vi "SCI_Rx_Pack.vi"(6 "确认":bool, 8 "SCI RX数据块":u16[](array[numeric]) format="%x") -> (3 "SciPckOut":T1={"包头"=170, "数据低8位"=0, "数据低高8位"=0, "数据类型"=0, "CRC余数"=0, "数据无效"=FALSE, "数据更新"=FALSE} {"包头" format="%02x"; "数据低8位" format="%02x"; "数据低高8位" format="%02x"; "数据类型" items=["VOID"]; "CRC余数" format="%02x"}, 5 "读数据块":u16[](array[numeric]) format="%x")   [LabVIEW 2015]
uses:
  SCI_DataPck.ctl
  SCI_DataType.ctl
  SCI_FrameIndex.ctl
  SCI_FrameNumber.ctl
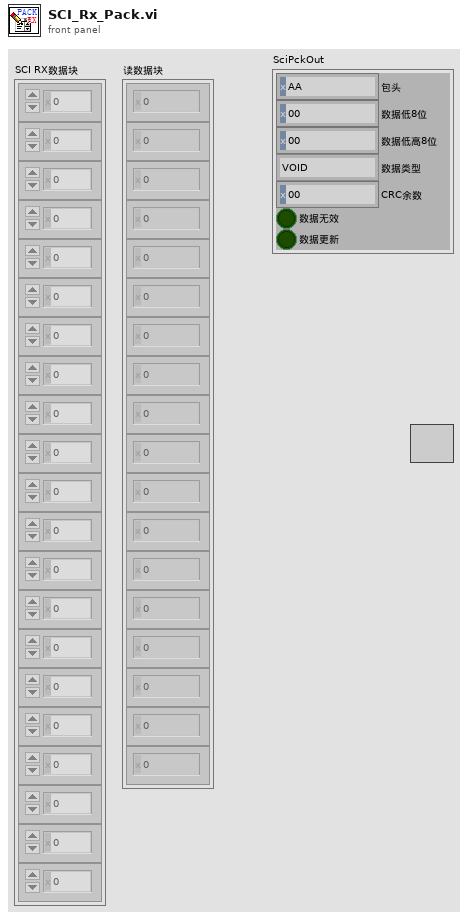
[diagram p1: front panel]
types:
  T1 = typedef "SCI_DataPck.ctl" = cluster{"包头":u16, "数据低8位":u16, "数据低高8位":u16, "数据类型":T2, "CRC余数":u16, "数据无效":bool, "数据更新":bool}
  T2 = typedef "SCI_DataType.ctl" = u16
  T3 = typedef "SCI_FrameNumber.ctl" = i32
  T4 = typedef "SCI_FrameIndex.ctl" = u16
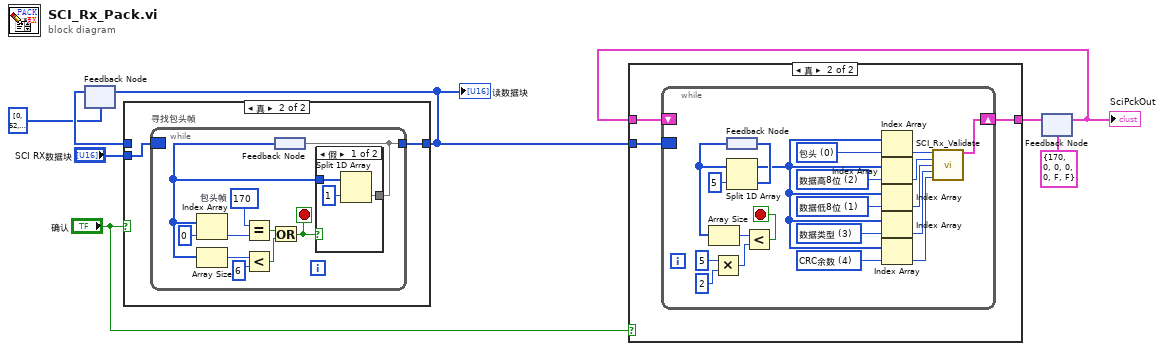
[diagram p0: block diagram]
diagram:
  n1 = feedback #1(u16[] [0, 52, 561, 35, 1075, 8, 0, 0, 0, 17, 14, 170, 801, 65535, 35, 170, 0, 1] ("数组 4")) -> (w8:u16[])
  n2 = case shown="真" "确认" {
    tunnel: [w9 w11] -> w6
    tunnel: w8 -> [w9 _]
    tunnel: "SCI RX数据块" -> [_ w10]
    frame False {
    }
    frame True {
      n3 = while "寻找包头帧" {
        tunnel: [w18] -> w11
        border: w10 -> [_]
        stop <- w12 stop-if-true
        w20 = u8 170  # 包头帧
        n4 = feedback #2() -> (w14:u16[])
        n5 = Index Array(array=w14, index=0) -> (element=w19:u16)
        n6 = Array Size(array=w14) -> (size(s)=w17:i32)
        n7 = Equal?(x=w20, y=w19) -> (x = y?=w13:bool)
        n8 = Less?(x=w17, y=6) -> (x < y?=w15:bool)
        n9 = Or(x=w13, y=w15) -> (x .or. y?=w12:bool)
        n10 = case shown="假" w12 {
          tunnel: w14 -> [w24 w25]
          tunnel: [w22 w25] -> w18
          frame False {
            n11 = Split 1D Array(array=w24, index=1) -> (second subarray=w22:u16[])  [unwired: 1 out]
          }
          frame True {
          }
        }
        n12 = feedback-in #2(w18) -> ()
      }
    }
  }
  "读数据块" <- w6
  n13 = feedback-in #1(w6) -> ()
  n14 = feedback #3(T1 {"包头"=170, "数据低8位"=0, "数据低高8位"=0, "数据类型"=0, "CRC余数"=0, "数据无效"=FALSE, "数据更新"=FALSE} ("SciPckOut")) -> (w2:T1)
  "SciPckOut" <- w2
  n15 = case shown="真" "确认" {
    tunnel: [w26 w28] -> w3
    tunnel: w6 -> [_ w29]
    tunnel: w2 -> [w26 w27]
    frame False {
    }
    frame True {
      n16 = while {
        border: w29 -> [_]
        shift-right: [w30] -> w28
        shift-left: w27 -> [_]
        stop <- w45 stop-if-true
        w39 = T4 4 items=["包头", "数据低8位", "数据高8位", "数据类型", "CRC余数"] ("帧索引")
        w40 = T4 3 items=["包头", "数据低8位", "数据高8位", "数据类型", "CRC余数"] ("帧索引")
        w43 = T4 1 items=["包头", "数据低8位", "数据高8位", "数据类型", "CRC余数"] ("帧索引")
        w42 = T4 2 items=["包头", "数据低8位", "数据高8位", "数据类型", "CRC余数"] ("帧索引")
        w41 = T4 0 items=["包头", "数据低8位", "数据高8位", "数据类型", "CRC余数"] ("帧索引")
        n17 = Multiply(x=T3 5 ("数值"), y=2) -> (x*y=w37:T3)
        n18 = feedback #4() -> (w47:u16[])
        n19 = Array Size(array=w47) -> (size(s)=w46:i32)
        n20 = Split 1D Array(array=w47, index=T3 5 ("数值")) -> (first subarray=w44:u16[], second subarray=w49:u16[])
        n21 = feedback-in #4(w49) -> ()
        n22 = Less?(x=w46, y=w37) -> (x < y?=w45:bool)
        n23 = Index Array(array=w44, index=w41) -> (element=w35:u16)
        n24 = Index Array(array=w44, index=w42) -> (element=w34:u16)
        n25 = Index Array(array=w44, index=w43) -> (element=w33:u16)
        n26 = Index Array(array=w44, index=w40) -> (element=w32:u16)
        n27 = Index Array(array=w44, index=w39) -> (element=w31:u16)
        n28 = call "SCI_Rx_Validate.vi"("Head"=w35, "Data8Hghr"=w34, "Data8Lwr"=w33, "Type"=w32, "CrcRsd"=w31) -> ("SciPckOut"=w30:T1)  [unwired: 10 in]
      }
    }
  }
  n29 = feedback-in #3(w3) -> ()
